vi "2.3.vi"() -> ()   [LabVIEW 2017]
uses:
  sin.vi
panel:
  out "一维数组":dbl[](array[numeric])
  out "转置":dbl[][](array[numeric])
  out "列数":dbl
  out "行数":dbl
  out "最小值":dbl
  out "最大值":dbl
  in  "数组":dbl[][](array[numeric])=[[12.0, 52.0, 89.0, 56.0], [2.0, 36.0, 45.0, 45.0], [10.0, 250.0, 850.0, 12.0]]
  in  "停止":bool
  # "任务三"
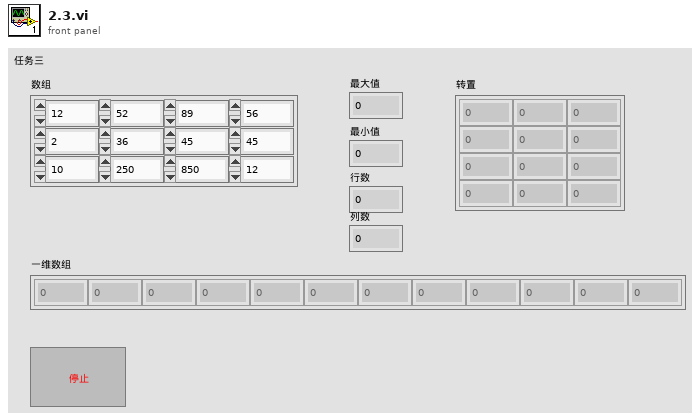
[diagram p1: front panel]
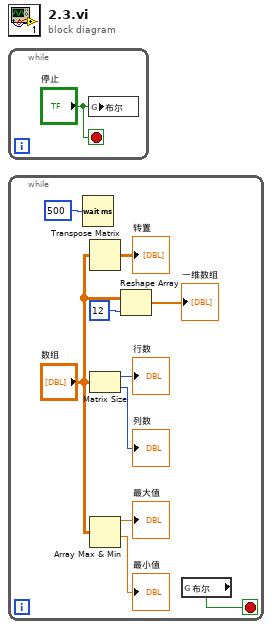
[diagram p0: block diagram]
diagram:
  n1 = while {
    stop <- "停止" stop-if-true
    n2 = global write "sin.vi" "布尔"("停止") -> ()
  }
  n3 = while {
    stop <- w9 stop-if-true
    n4 = Wait (ms)(milliseconds to wait=500) -> ()  [unwired: 1 out]
    n5 = Transpose Matrix(1:"数组") -> (0:→"转置":dbl[][])
    n6 = Matrix Size(0:"数组") -> (1:→"行数":i32, 2:→"列数":i32)
    n7 = Array Max & Min(array="数组") -> (max value=→"最大值":dbl, min value=→"最小值":dbl)  [unwired: 2 out]
    n8 = Reshape Array("数组", 12) -> (→"一维数组":dbl[])
    n9 = global read "sin.vi" "布尔"() -> (w9:bool)
  }
